vi "FilecsvOpen.vi"(6 "提示语":refnum<vi>, 7 "Language":u32, 8 "进度条":refnum<vi>, 9 "进度数值":refnum<vi>, 10 "报文行数统计":refnum<vi>, 11 "file path (dialog if empty)":path caption="文件路径 （空时为对话框）") -> (0 "路径输出":path, 1 "重构的Data数组":u32[][](array[numeric]), 2 "统计数量":string[](array[string]), 3 "报文ID":string[](array[string]), 4 "基时间簇":T1, 5 "CAN报文统计":string[][](array[string]))   [LabVIEW 2015]
uses:
  <vilib>/Utility/file.llb/Read Delimited Spreadsheet (string).vi
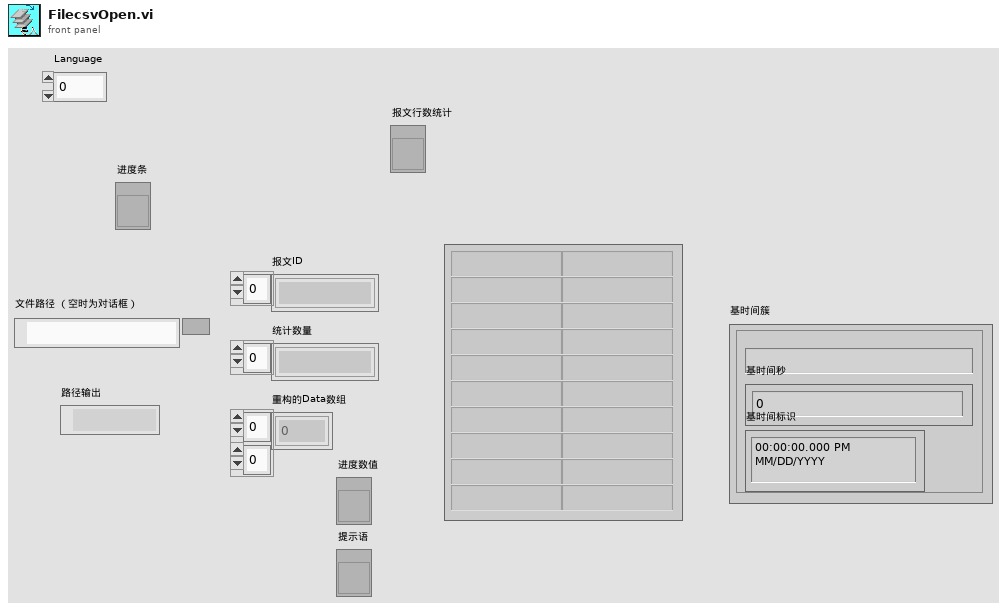
[diagram p1: front panel]
types:
  T1 = cluster{"基时间字符串":string, "基时间秒":dbl, "基时间标识":timestamp}
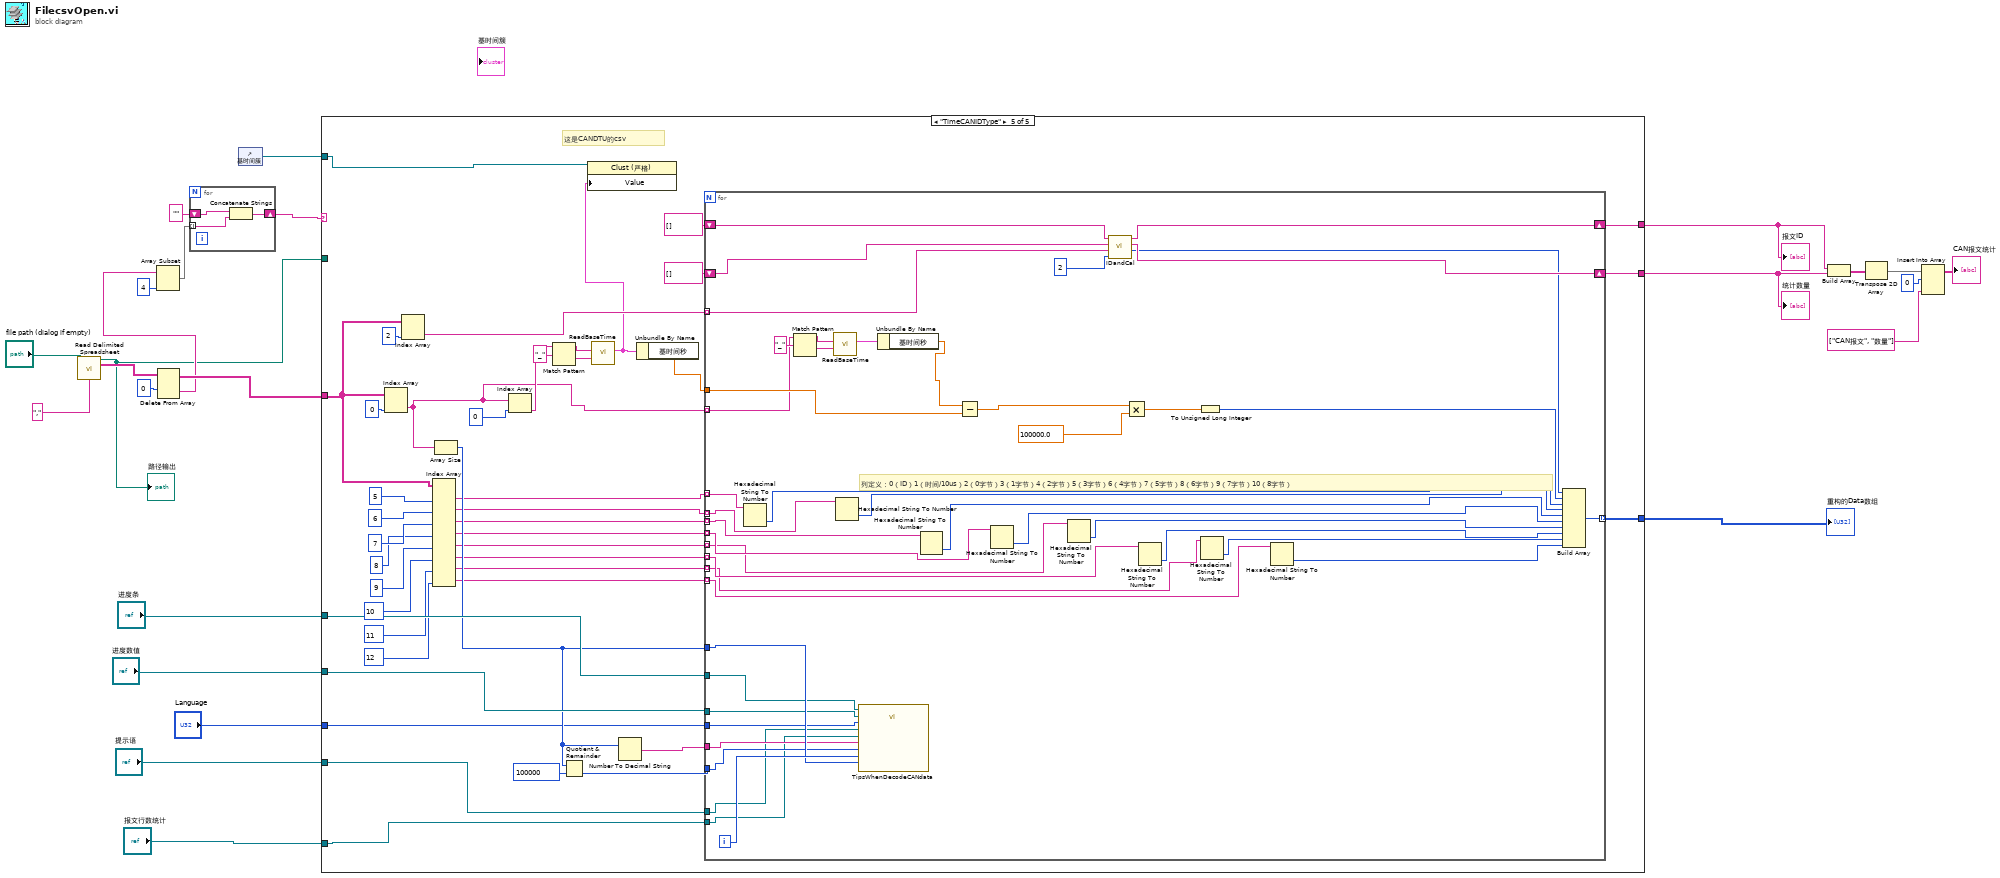
[diagram p0: block diagram]
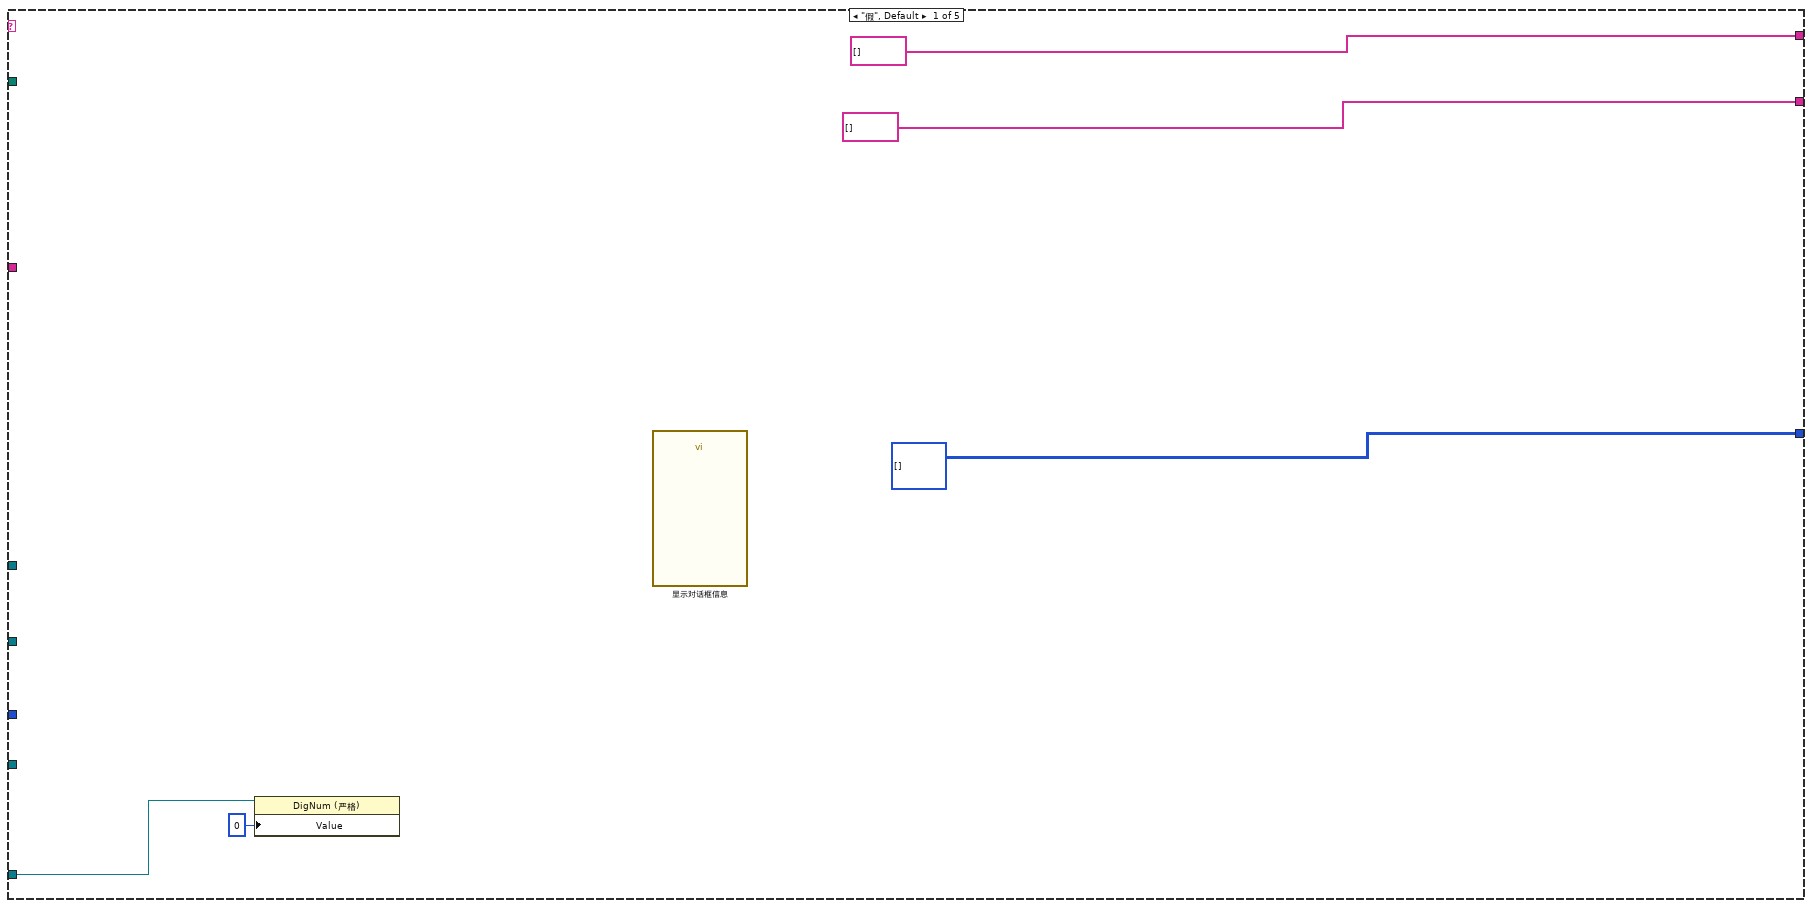
[diagram p2: hidden frame]
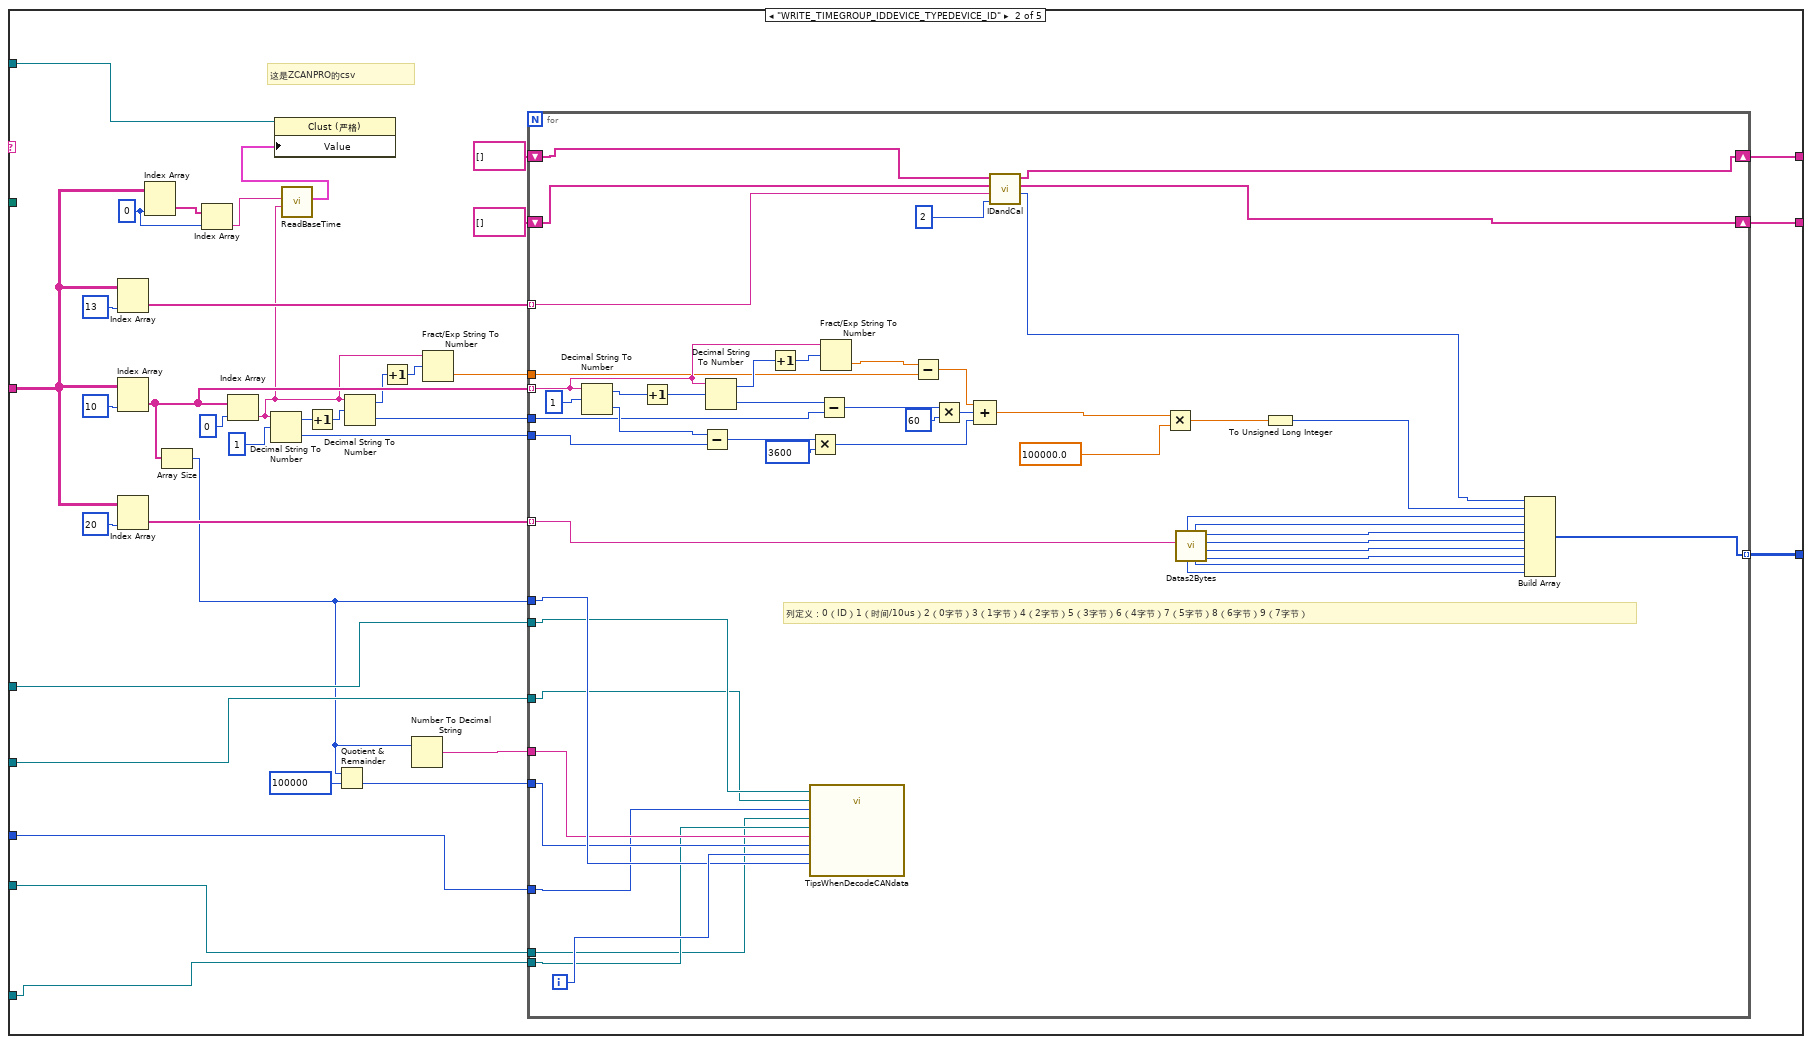
[diagram p3: hidden frame]
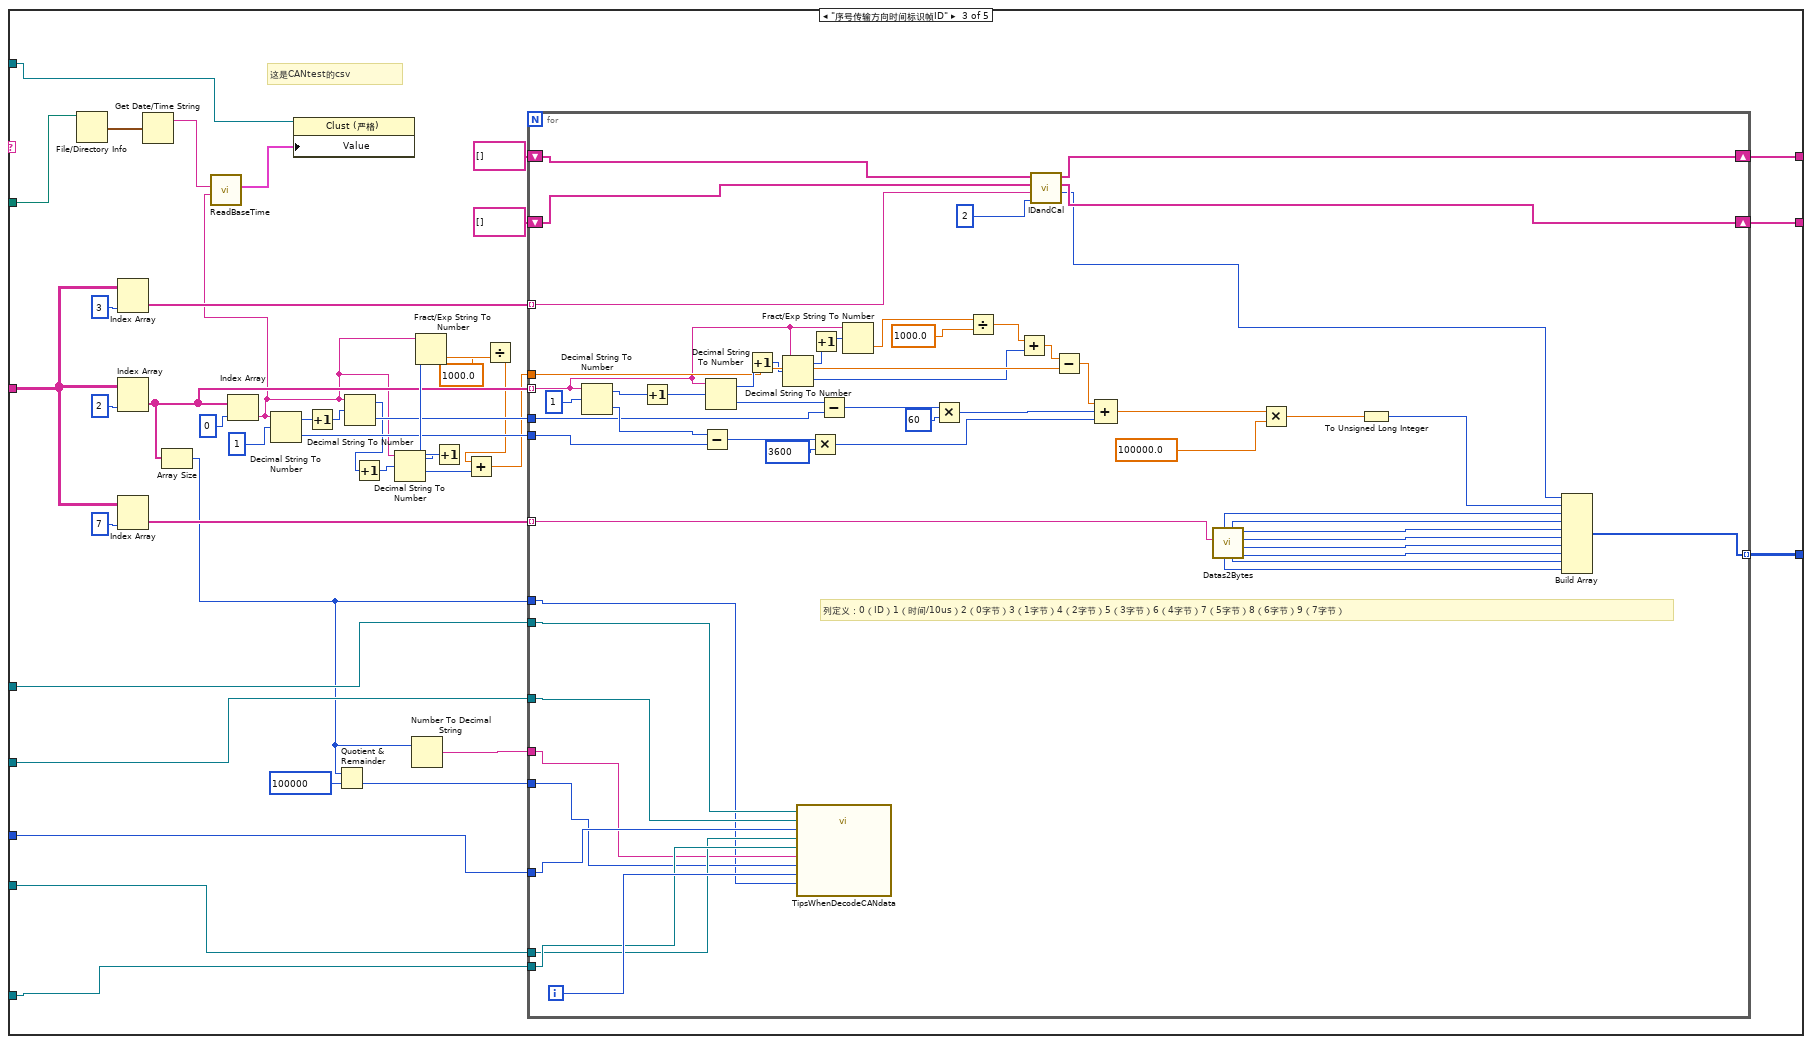
[diagram p4: hidden frame]
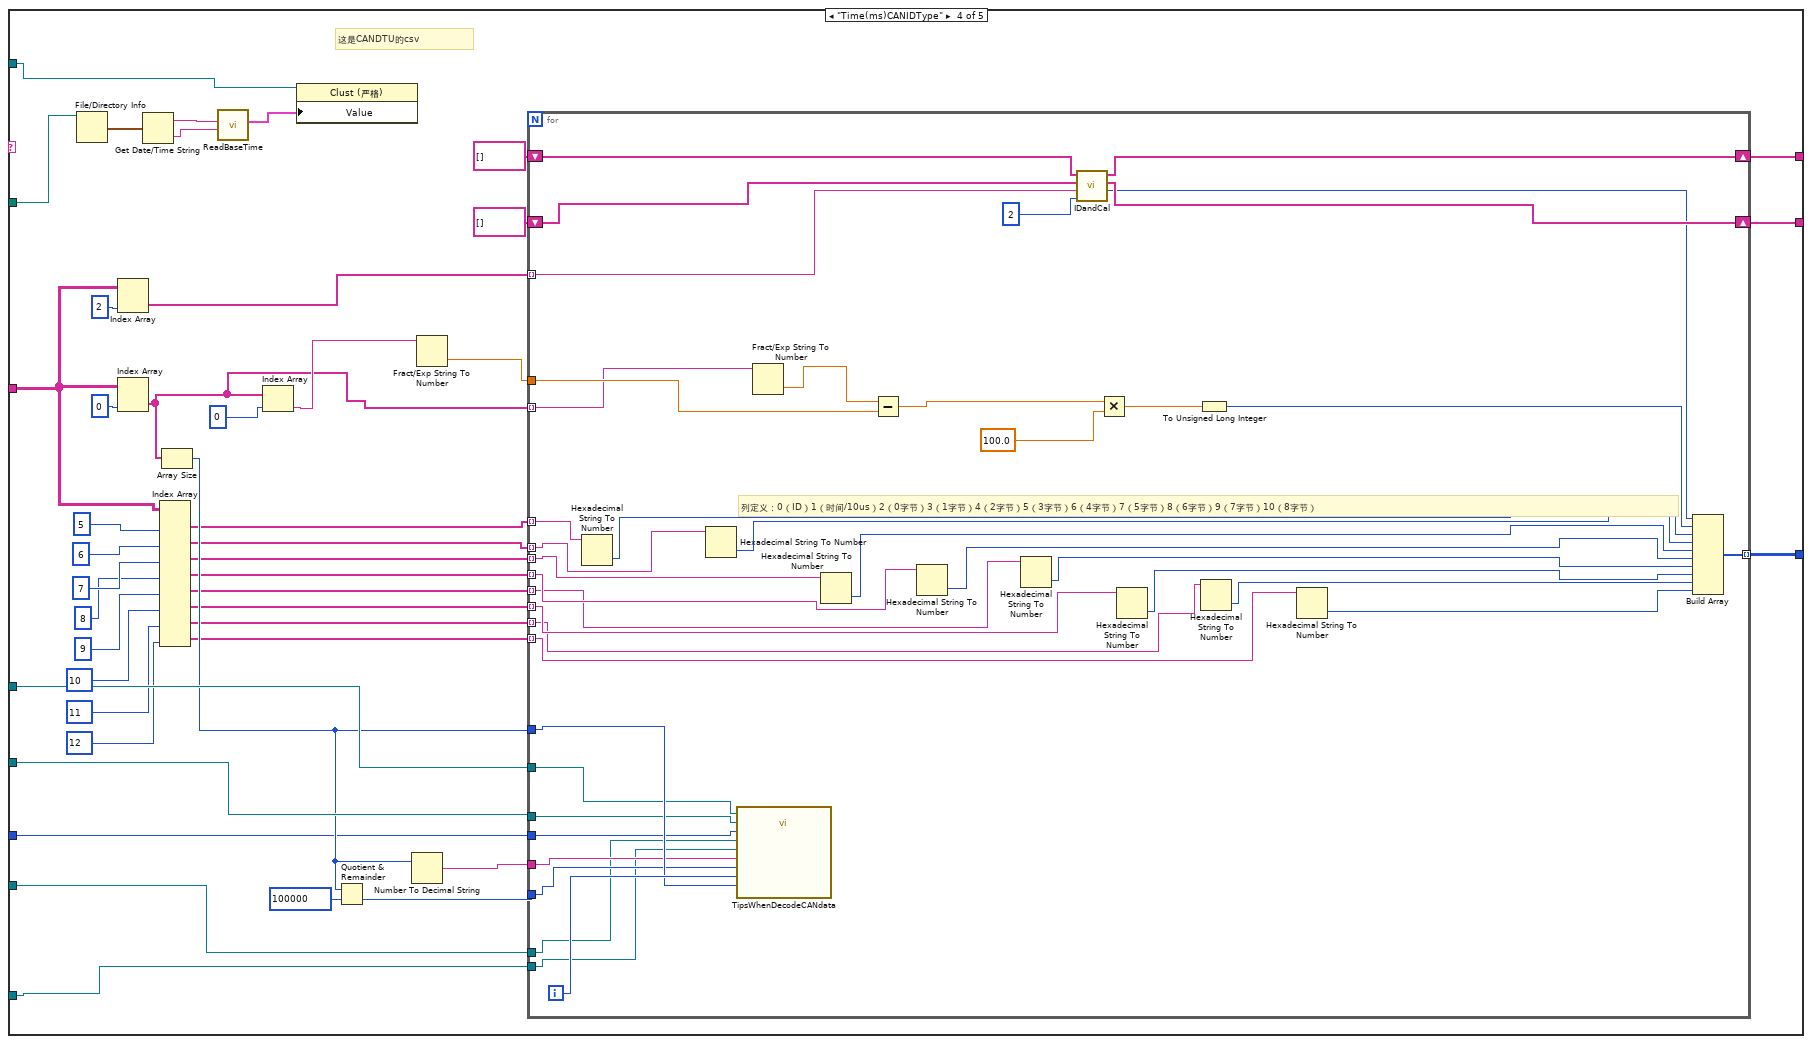
[diagram p5: hidden frame]
diagram:
  n1 = call-poly <vilib>:"Read Delimited Spreadsheet.vi"("file path (dialog if empty)"="file path (dialog if empty)", "delimiter (\\t)"="," ("delimiter (\\t)")) -> ("new file path (Not A Path if cancelled)"=w1:path, "all rows"=w15:string[][])  [unwired: 8 in, 4 out]
  "路径输出" <- w1
  n2 = Delete From Array(array=w15, index (row)=0 ("索引 (行)")) -> (deleted portion=w5:string[], array with subset deleted=w24:string[][])  [unwired: 2 in]
  n3 = Array Subset(array=w5, length=4 ("长度")) -> (w6:string[])  [unwired: 1 in]
  n4 = for {
    tunnel: w6 -> [w27] mode=indexing
    shift-right: [w28] -> w8
    shift-left: "" -> [w26]
    n5 = Concatenate Strings(w26, w27) -> (w28:string)
  }
  n6 = control-ref of="基时间簇"() -> (w3:refnum<vi>)
  n7 = case shown="\"TimeCANIDType\"" w8 {
    tunnel: [u32[][] [] w69 w160 w259 w342] -> w25
    tunnel: w24 -> [_ w41 w158 w226 w318]
    tunnel: [string[] [] w52 w144 w253 w337] -> w18
    tunnel: [string[] [] w51 w143 w252 w336] -> w17
    tunnel: "进度条" -> [_ w50 w142 w251 w335]
    tunnel: "进度数值" -> [_ w49 w141 w250 w334]
    tunnel: "提示语" -> [_ w36 w138 w247 w331]
    tunnel: "报文行数统计" -> [w30 w35 w120 w239 w327]
    tunnel: w3 -> [_ w38 w122 w241 w328]
    tunnel: w1 -> [_ _ w125 w243 _]
    tunnel: "Language" -> [_ w34 w119 w216 w308]
    frame "假", Default {
      n8 = property class="DigNum (严格)"(reference=w30, "Value"=0 ("值")) -> ()  [unwired: 1 in, 2 out]
      n9 = call "显示对话框信息"() -> ()  [unwired: 10 in, 2 out]
    }
    frame "WRITE_TIMEGROUP_IDDEVICE_TYPEDEVICE_ID" {
      w42 = 0 ("禁用的索引 (列)")
      # "这是ZCANPRO的csv"
      n10 = Index Array(array=w41, index (col)=13 ("禁用的索引 (列)")) -> (element=w68:string[])  [unwired: 1 in]
      n11 = Index Array(array=w41, index (col)=10 ("禁用的索引 (列)")) -> (element=w59:string[])  [unwired: 1 in]
      n12 = Index Array(array=w41, index (col)=20 ("禁用的索引 (列)")) -> (element=w64:string[])  [unwired: 1 in]
      n13 = Index Array(array=w41, index (col)=w42) -> (element=w43:string[])  [unwired: 1 in]
      n14 = Array Size(array=w59) -> (size(s)=w45:i32)
      n15 = Index Array(array=w43, index=w42) -> (element=w40:string)
      n16 = Index Array(array=w59, index=0 ("索引")) -> (element=w39:string)
      n17 = Decimal String To Number(string=w39, offset=1 ("偏移量")) -> (offset past number=w56:i32, number=w60:i32)  [unwired: 1 in]
      n18 = call "ReadBaseTime.vi"("时间字符"=w39, "日期字符"=w40) -> ("基时间簇"=w37:T1)  [unwired: 7 in]
      n19 = property class="Clust (严格)"(reference=w38, "Value"=w37) -> ()  [unwired: 1 in, 2 out]
      n20 = Increment(x=w56) -> (x+1=w57:i32)
      n21 = Quotient & Remainder(x=w45, y=100000) -> (floor(x/y)=w47:i32)  [unwired: 1 out]
      n22 = Decimal String To Number(string=w39, offset=w57) -> (offset past number=w58:i32, number=w61:i32)  [unwired: 1 in]
      n23 = Increment(x=w58) -> (x+1=w62:i32)
      n24 = Number To Decimal String(number=w45) -> (decimal integer string=w46:string)  [unwired: 1 in]
      n25 = Fract/Exp String To Number(string=w39, offset=w62) -> (number=w63:dbl)  [unwired: 2 in, 1 out]
      n26 = for {
        tunnel: w59 -> [w104] mode=indexing
        tunnel: w60 -> [w114]
        tunnel: w61 -> [w110]
        tunnel: w63 -> [w102]
        tunnel: w64 -> [w70] mode=indexing
        tunnel: [w73] -> w69 mode=indexing
        shift-right: [w86] -> w52
        shift-left: string[] [] -> [w84]
        shift-right: [w85] -> w51
        shift-left: string[] [] -> [w83]
        tunnel: w68 -> [w82] mode=indexing
        tunnel: w45 -> [w95]
        tunnel: w50 -> [w94]
        tunnel: w49 -> [w93]
        tunnel: w47 -> [w92]
        tunnel: w36 -> [w89]
        tunnel: w46 -> [w91]
        tunnel: w35 -> [w90]
        tunnel: w34 -> [w88]
        i -> [w96]
        # "列定义：0（ID）1（时间/10us）2（0字节）3（1字节）4（2字节）5（3字节）6（4字节）7（5字节）8（6字节）9（7字节）"
        n27 = Decimal String To Number(string=w104, offset=1 ("偏移量")) -> (offset past number=w116:i32, number=w115:i32)  [unwired: 1 in]
        n28 = Increment(x=w116) -> (x+1=w117:i32)
        n29 = Subtract(x=w115, y=w114) -> (x-y=w113:i32)
        n30 = Decimal String To Number(string=w104, offset=w117) -> (offset past number=w118:i32, number=w111:i32)  [unwired: 1 in]
        n31 = Increment(x=w118) -> (x+1=w105:i32)
        n32 = Multiply(x=w113, y=3600) -> (x*y=w106:i32)
        n33 = call "TipsWhenDecodeCANdata.vi"("ProgressBar"=w94, "AllRowsNum"=w95, "i"=w96, "ProgressNum"=w93, "Language"=w88, "Tips"=w89, "MessageLinCnt"=w90, "txtAllRowsNum"=w91, "RowsLevel"=w92) -> ()  [unwired: 7 in]
        n34 = Subtract(x=w111, y=w110) -> (x-y=w109:i32)
        n35 = Fract/Exp String To Number(string=w104, offset=w105) -> (number=w103:dbl)  [unwired: 2 in, 1 out]
        n36 = Subtract(x=w103, y=w102) -> (x-y=w101:dbl)
        n37 = Multiply(x=w109, y=60) -> (x*y=w107:i32)
        n38 = Compound Arithmetic op=ADD(w101, w107, w106) -> (w100:dbl)
        n39 = call "IDandCal.vi"("ID列表In"=w84, "数量统计in"=w83, "ID输入"=w82, "偏移量(0)"=2) -> ("ID列表"=w86:string[], "数量统计"=w85:string[], "ID输出"=w72:u32)  [unwired: 3 in]
        n40 = Multiply(x=w100, y=100000.0) -> (x*y=w98:dbl)
        n41 = call "Datas2Bytes.vi"("DATAs"=w70) -> ("Data5"=w76:u32, "Data4"=w77:u32, "Data3"=w78:u32, "Data2"=w79:u32, "Data6"=w75:u32, "Data1"=w80:u32, "Data7"=w74:u32, "Data0"=w81:u32)  [unwired: 3 in]
        n42 = To Unsigned Long Integer(number=w98) -> (unsigned 32bit integer=w71:u32)
        n43 = Build Array(w72, w71, w81, w80, w79, w78, w77, w76, w75, w74) -> (w73:u32[])
      }
    }
    frame "序号传输方向时间标识帧ID" {
      # "这是CANtest的csv"
      n44 = File/Directory Info(path=w125) -> (last mod=w126:timestamp)  [unwired: 1 in, 6 out]
      n45 = Index Array(array=w158, index (col)=3 ("禁用的索引 (列)")) -> (element=w159:string[])  [unwired: 1 in]
      n46 = Index Array(array=w158, index (col)=2 ("禁用的索引 (列)")) -> (element=w150:string[])  [unwired: 1 in]
      n47 = Index Array(array=w158, index (col)=7 ("禁用的索引 (列)")) -> (element=w154:string[])  [unwired: 1 in]
      n48 = Get Date/Time String(seconds (now)=w126) -> (date string=w124:string)  [unwired: 2 in, 1 out]
      n49 = Array Size(array=w150) -> (size(s)=w136:i32)
      n50 = Index Array(array=w150, index=0 ("索引")) -> (element=w123:string)
      n51 = call "ReadBaseTime.vi"("时间字符"=w123, "日期字符"=w124) -> ("基时间簇"=w121:T1)  [unwired: 7 in]
      n52 = Decimal String To Number(string=w123, offset=1 ("偏移量")) -> (offset past number=w148:i32, number=w151:i32)  [unwired: 1 in]
      n53 = property class="Clust (严格)"(reference=w122, "Value"=w121) -> ()  [unwired: 1 in, 2 out]
      n54 = Increment(x=w148) -> (x+1=w149:i32)
      n55 = Quotient & Remainder(x=w136, y=100000) -> (floor(x/y)=w139:i32)  [unwired: 1 out]
      n56 = Decimal String To Number(string=w123, offset=w149) -> (offset past number=w133:i32, number=w152:i32)  [unwired: 1 in]
      n57 = Increment(x=w133) -> (x+1=w134:i32)
      n58 = Decimal String To Number(string=w123, offset=w134) -> (offset past number=w131:i32, number=w132:i32)  [unwired: 1 in]
      n59 = Number To Decimal String(number=w136) -> (decimal integer string=w137:string)  [unwired: 1 in]
      n60 = Increment(x=w131) -> (x+1=w153:i32)
      n61 = Fract/Exp String To Number(string=w123, offset=w153) -> (number=w128:dbl)  [unwired: 2 in, 1 out]
      n62 = Divide(x=w128, y=1000.0) -> (x/y=w129:dbl)
      n63 = Add(x=w129, y=w132) -> (x+y=w130:dbl)
      n64 = for {
        tunnel: w150 -> [w193] mode=indexing
        tunnel: w151 -> [w211]
        tunnel: w152 -> [w207]
        tunnel: w130 -> [w202]
        tunnel: w154 -> [w161] mode=indexing
        tunnel: [w164] -> w160 mode=indexing
        shift-right: [w177] -> w144
        shift-left: string[] [] -> [w173]
        shift-right: [w176] -> w143
        shift-left: string[] [] -> [w174]
        tunnel: w159 -> [w175] mode=indexing
        tunnel: w136 -> [w179]
        tunnel: w142 -> [w186]
        tunnel: w141 -> [w182]
        tunnel: w139 -> [w180]
        tunnel: w138 -> [w184]
        tunnel: w137 -> [w181]
        tunnel: w120 -> [w185]
        tunnel: w119 -> [w183]
        i -> [w187]
        # "列定义：0（ID）1（时间/10us）2（0字节）3（1字节）4（2字节）5（3字节）6（4字节）7（5字节）8（6字节）9（7字节）"
        n65 = Decimal String To Number(string=w193, offset=1 ("偏移量")) -> (offset past number=w213:i32, number=w212:i32)  [unwired: 1 in]
        n66 = Increment(x=w213) -> (x+1=w214:i32)
        n67 = Subtract(x=w212, y=w211) -> (x-y=w210:i32)
        n68 = Decimal String To Number(string=w193, offset=w214) -> (offset past number=w215:i32, number=w208:i32)  [unwired: 1 in]
        n69 = Increment(x=w215) -> (x+1=w194:i32)
        n70 = Decimal String To Number(string=w193, offset=w194) -> (offset past number=w192:i32, number=w191:i32)  [unwired: 1 in]
        n71 = call "TipsWhenDecodeCANdata.vi"("ProgressBar"=w186, "AllRowsNum"=w179, "i"=w187, "ProgressNum"=w182, "Language"=w183, "Tips"=w184, "MessageLinCnt"=w185, "txtAllRowsNum"=w181, "RowsLevel"=w180) -> ()  [unwired: 7 in]
        n72 = Multiply(x=w210, y=3600) -> (x*y=w203:i32)
        n73 = Increment(x=w192) -> (x+1=w195:i32)
        n74 = Subtract(x=w208, y=w207) -> (x-y=w206:i32)
        n75 = Fract/Exp String To Number(string=w193, offset=w195) -> (number=w190:dbl)  [unwired: 2 in, 1 out]
        n76 = Multiply(x=w206, y=60) -> (x*y=w204:i32)
        n77 = Divide(x=w190, y=1000.0) -> (x/y=w188:dbl)
        n78 = Add(x=w188, y=w191) -> (x+y=w196:dbl)
        n79 = call "IDandCal.vi"("ID列表In"=w173, "数量统计in"=w174, "ID输入"=w175, "偏移量(0)"=2) -> ("ID列表"=w177:string[], "数量统计"=w176:string[], "ID输出"=w163:u32)  [unwired: 3 in]
        n80 = Subtract(x=w196, y=w202) -> (x-y=w201:dbl)
        n81 = Compound Arithmetic op=ADD(w201, w204, w203) -> (w200:dbl)
        n82 = call "Datas2Bytes.vi"("DATAs"=w161) -> ("Data5"=w167:u32, "Data4"=w168:u32, "Data3"=w169:u32, "Data2"=w170:u32, "Data6"=w166:u32, "Data1"=w171:u32, "Data7"=w165:u32, "Data0"=w172:u32)  [unwired: 3 in]
        n83 = Multiply(x=w200, y=100000.0) -> (x*y=w198:dbl)
        n84 = To Unsigned Long Integer(number=w198) -> (unsigned 32bit integer=w162:u32)
        n85 = Build Array(w163, w162, w172, w171, w170, w169, w168, w167, w166, w165) -> (w164:u32[])
      }
    }
    frame "Time(ms)CANIDType" {
      # "这是CANDTU的csv"
      n86 = File/Directory Info(path=w243) -> (last mod=w244:timestamp)  [unwired: 1 in, 6 out]
      n87 = Index Array(array=w226, index (col)=2 ("禁用的索引 (列)")) -> (element=w258:string[])  [unwired: 1 in]
      n88 = Index Array(array=w226, index (col)=0 ("禁用的索引 (列)")) -> (element=w234:string[])  [unwired: 1 in]
      n89 = Get Date/Time String(seconds (now)=w244) -> (date string=w242:string, time string=w238:string)  [unwired: 2 in]
      n90 = Index Array(array=w226, index (col) #1=5 ("禁用的索引 (列)"), index (col) #2=6 ("禁用的索引 (列)"), index (col) #3=7 ("禁用的索引 (列)"), index (col) #4=8 ("禁用的索引 (列)"), index (col) #5=9 ("禁用的索引 (列)"), index (col) #6=10 ("禁用的索引 (列)"), index (col) #7=11 ("禁用的索引 (列)"), index (col) #8=12 ("禁用的索引 (列)")) -> (element #1=w225:string[], element #2=w223:string[], element #3=w222:string[], element #4=w221:string[], element #5=w220:string[], element #6=w219:string[], element #7=w218:string[], element #8=w217:string[])  [unwired: 8 in]
      n91 = Array Size(array=w234) -> (size(s)=w245:i32)
      n92 = call "ReadBaseTime.vi"("时间字符"=w238, "日期字符"=w242) -> ("基时间簇"=w240:T1)  [unwired: 7 in]
      n93 = Index Array(array=w234, index=0 ("索引")) -> (element=w236:string)
      n94 = property class="Clust (严格)"(reference=w241, "Value"=w240) -> ()  [unwired: 1 in, 2 out]
      n95 = Quotient & Remainder(x=w245, y=100000) -> (floor(x/y)=w248:i32)  [unwired: 1 out]
      n96 = Number To Decimal String(number=w245) -> (decimal integer string=w246:string)  [unwired: 1 in]
      n97 = Fract/Exp String To Number(string=w236) -> (number=w235:dbl)  [unwired: 3 in, 1 out]
      n98 = for {
        tunnel: w225 -> [w287] mode=indexing
        tunnel: [w291] -> w259 mode=indexing
        shift-right: [w266] -> w253
        shift-left: string[] [] -> [w260]
        shift-right: [w265] -> w252
        shift-left: string[] [] -> [w261]
        tunnel: w258 -> [w262] mode=indexing
        tunnel: w245 -> [w274]
        tunnel: w251 -> [w267]
        tunnel: w250 -> [w268]
        tunnel: w248 -> [w273]
        tunnel: w247 -> [w270]
        tunnel: w246 -> [w272]
        tunnel: w239 -> [w271]
        tunnel: w235 -> [w285]
        tunnel: w234 -> [w284] mode=indexing
        tunnel: w223 -> [w282] mode=indexing
        tunnel: w222 -> [w281] mode=indexing
        tunnel: w221 -> [w280] mode=indexing
        tunnel: w220 -> [w279] mode=indexing
        tunnel: w219 -> [w278] mode=indexing
        tunnel: w218 -> [w277] mode=indexing
        tunnel: w217 -> [w276] mode=indexing
        tunnel: w216 -> [w269]
        i -> [w275]
        # "列定义：0（ID）1（时间/10us）2（0字节）3（1字节）4（2字节）5（3字节）6（4字节）7（5字节）8（6字节）9（7字节）10（8字节）"
        n99 = Hexadecimal String To Number(string=w287) -> (number=w299:u32)  [unwired: 2 in, 1 out]
        n100 = Hexadecimal String To Number(string=w282) -> (number=w298:u32)  [unwired: 2 in, 1 out]
        n101 = call "TipsWhenDecodeCANdata.vi"("ProgressBar"=w267, "AllRowsNum"=w274, "i"=w275, "ProgressNum"=w268, "Language"=w269, "Tips"=w270, "MessageLinCnt"=w271, "txtAllRowsNum"=w272, "RowsLevel"=w273) -> ()  [unwired: 7 in]
        n102 = Fract/Exp String To Number(string=w284) -> (number=w286:dbl)  [unwired: 3 in, 1 out]
        n103 = Hexadecimal String To Number(string=w281) -> (number=w297:u32)  [unwired: 2 in, 1 out]
        n104 = Subtract(x=w286, y=w285) -> (x-y=w283:dbl)
        n105 = Hexadecimal String To Number(string=w280) -> (number=w296:u32)  [unwired: 2 in, 1 out]
        n106 = Hexadecimal String To Number(string=w279) -> (number=w295:u32)  [unwired: 2 in, 1 out]
        n107 = call "IDandCal.vi"("ID列表In"=w260, "数量统计in"=w261, "ID输入"=w262, "偏移量(0)"=2) -> ("ID列表"=w266:string[], "数量统计"=w265:string[], "ID输出"=w264:u32)  [unwired: 3 in]
        n108 = Multiply(x=w283, y=100.0) -> (x*y=w289:dbl)
        n109 = Hexadecimal String To Number(string=w278) -> (number=w294:u32)  [unwired: 2 in, 1 out]
        n110 = To Unsigned Long Integer(number=w289) -> (unsigned 32bit integer=w288:u32)
        n111 = Hexadecimal String To Number(string=w277) -> (number=w293:u32)  [unwired: 2 in, 1 out]
        n112 = Hexadecimal String To Number(string=w276) -> (number=w292:u32)  [unwired: 2 in, 1 out]
        n113 = Build Array(w264, w288, w299, w298, w297, w296, w295, w294, w293, w292) -> (w291:u32[])
      }
    }
    frame "TimeCANIDType" {
      # "这是CANDTU的csv"
      n114 = Index Array(array=w318, index (col)=0 ("禁用的索引 (列)")) -> (element=w301:string[])  [unwired: 1 in]
      n115 = Index Array(array=w318, index (col)=2 ("禁用的索引 (列)")) -> (element=w341:string[])  [unwired: 1 in]
      n116 = Index Array(array=w318, index (col) #1=5 ("禁用的索引 (列)"), index (col) #2=6 ("禁用的索引 (列)"), index (col) #3=7 ("禁用的索引 (列)"), index (col) #4=8 ("禁用的索引 (列)"), index (col) #5=9 ("禁用的索引 (列)"), index (col) #6=10 ("禁用的索引 (列)"), index (col) #7=11 ("禁用的索引 (列)"), index (col) #8=12 ("禁用的索引 (列)")) -> (element #1=w317:string[], element #2=w315:string[], element #3=w314:string[], element #4=w313:string[], element #5=w312:string[], element #6=w311:string[], element #7=w310:string[], element #8=w309:string[])  [unwired: 8 in]
      n117 = Array Size(array=w301) -> (size(s)=w329:i32)
      n118 = Index Array(array=w301, index=0 ("索引")) -> (element=w306:string)
      n119 = Match Pattern(string=w306, regular expression="_" ("正则表达式")) -> (before substring=w305:string, after substring=w304:string)  [unwired: 1 in, 2 out]
      n120 = Quotient & Remainder(x=w329, y=100000) -> (floor(x/y)=w332:i32)  [unwired: 1 out]
      n121 = call "ReadBaseTime.vi"("时间字符"=w304, "日期字符"=w305) -> ("基时间簇"=w300:T1)  [unwired: 7 in]
      n122 = property class="Clust (严格)"(reference=w328, "Value"=w300) -> ()  [unwired: 1 in, 2 out]
      n123 = Number To Decimal String(number=w329) -> (decimal integer string=w330:string)  [unwired: 1 in]
      n124 = Unbundle By Name(w300) -> ("基时间秒"=w303:dbl)
      n125 = for {
        tunnel: w317 -> [w374] mode=indexing
        tunnel: [w378] -> w342 mode=indexing
        shift-right: [w355] -> w337
        shift-left: string[] [] -> [w349]
        shift-right: [w354] -> w336
        shift-left: string[] [] -> [w350]
        tunnel: w341 -> [w351] mode=indexing
        tunnel: w329 -> [w363]
        tunnel: w335 -> [w356]
        tunnel: w334 -> [w357]
        tunnel: w332 -> [w362]
        tunnel: w331 -> [w359]
        tunnel: w330 -> [w361]
        tunnel: w327 -> [w360]
        tunnel: w303 -> [w373]
        tunnel: w301 -> [w344] mode=indexing
        tunnel: w315 -> [w371] mode=indexing
        tunnel: w314 -> [w370] mode=indexing
        tunnel: w313 -> [w369] mode=indexing
        tunnel: w312 -> [w368] mode=indexing
        tunnel: w311 -> [w367] mode=indexing
        tunnel: w310 -> [w366] mode=indexing
        tunnel: w309 -> [w365] mode=indexing
        tunnel: w308 -> [w358]
        i -> [w364]
        # "列定义：0（ID）1（时间/10us）2（0字节）3（1字节）4（2字节）5（3字节）6（4字节）7（5字节）8（6字节）9（7字节）10（8字节）"
        n126 = Hexadecimal String To Number(string=w374) -> (number=w386:u32)  [unwired: 2 in, 1 out]
        n127 = Match Pattern(string=w344, regular expression="_" ("正则表达式")) -> (before substring=w347:string, after substring=w346:string)  [unwired: 1 in, 2 out]
        n128 = call "ReadBaseTime.vi"("时间字符"=w346, "日期字符"=w347) -> ("基时间簇"=w345:T1)  [unwired: 7 in]
        n129 = Hexadecimal String To Number(string=w371) -> (number=w385:u32)  [unwired: 2 in, 1 out]
        n130 = call "TipsWhenDecodeCANdata.vi"("ProgressBar"=w356, "AllRowsNum"=w363, "i"=w364, "ProgressNum"=w357, "Language"=w358, "Tips"=w359, "MessageLinCnt"=w360, "txtAllRowsNum"=w361, "RowsLevel"=w362) -> ()  [unwired: 7 in]
        n131 = Unbundle By Name(w345) -> ("基时间秒"=w343:dbl)
        n132 = Hexadecimal String To Number(string=w370) -> (number=w384:u32)  [unwired: 2 in, 1 out]
        n133 = Subtract(x=w343, y=w373) -> (x-y=w372:dbl)
        n134 = Hexadecimal String To Number(string=w369) -> (number=w383:u32)  [unwired: 2 in, 1 out]
        n135 = Hexadecimal String To Number(string=w368) -> (number=w382:u32)  [unwired: 2 in, 1 out]
        n136 = call "IDandCal.vi"("ID列表In"=w349, "数量统计in"=w350, "ID输入"=w351, "偏移量(0)"=2) -> ("ID列表"=w355:string[], "数量统计"=w354:string[], "ID输出"=w353:u32)  [unwired: 3 in]
        n137 = Multiply(x=w372, y=100000.0) -> (x*y=w376:dbl)
        n138 = Hexadecimal String To Number(string=w367) -> (number=w381:u32)  [unwired: 2 in, 1 out]
        n139 = To Unsigned Long Integer(number=w376) -> (unsigned 32bit integer=w375:u32)
        n140 = Hexadecimal String To Number(string=w366) -> (number=w380:u32)  [unwired: 2 in, 1 out]
        n141 = Hexadecimal String To Number(string=w365) -> (number=w379:u32)  [unwired: 2 in, 1 out]
        n142 = Build Array(w353, w375, w386, w385, w384, w383, w382, w381, w380, w379) -> (w378:u32[])
      }
    }
  }
  "重构的Data数组" <- w25
  "报文ID" <- w18
  "统计数量" <- w17
  n143 = Build Array(w18, w17) -> (w22:string[][])
  n144 = Transpose 2D Array(2D array=w22) -> (transposed array=w21:string[][])
  n145 = Insert Into Array(array=w21, index (row)=0 ("索引 (行)"), new element=string[] ["CAN报文", "数量"]) -> (→"CAN报文统计":string[][])  [unwired: 1 in]
